vi "AutoWait.vi"(8 "error in (no error)":errorcluster, 11 "TimeOut (s)":dbl) -> (0 "error out":errorcluster)   [LabVIEW 2023]
doc: "Wrapper class for auto do nothing and wait\nInput:\n -- error in -- Cluster \n -- time out -- Double -- how long to wait B4 quitting\nOutput:\n -- error out -- Cluster"
uses:
  <vilib>/Rock Robotics/WPI/ThirdParty/JAS_Junk/TrajLib/ChassisSpeeds_New.vi
  <vilib>/Rock Robotics/WPI/ThirdParty/JAS_Junk/TrajLib/Conv_Feet_Meters.vi
  <vilib>/Rock Robotics/WPI/ThirdParty/JAS_Junk/TrajLib/Conv_Deg_Radians.vi
  <vilib>/Utility/semaphor.llb/Obtain Semaphore Reference.vi
  <vilib>/Rock Robotics/WPI/ThirdParty/JAS_Junk/TrajLib/Timer_Reset.vi
  Drive/DriveGlobal.vi
  <vilib>/Rock Robotics/WPI/ThirdParty/JAS_Junk/TrajLib/Trajectory_Library.lvlib
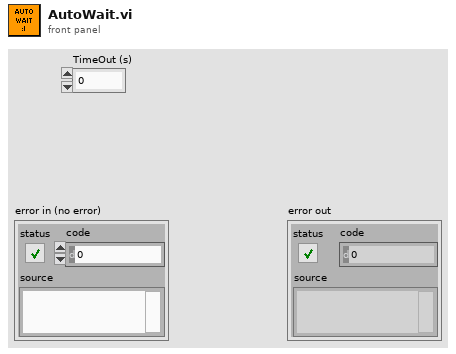
[diagram p1: front panel]
types:
  T1 = typedef "Trajectory_Library.lvlib/TIMER.ctl" = cluster{"StartTime":dbl, "Accumulated TIme":dbl, "Running":bool, "semaphore":T2}
  T2 = typedef "Semaphore RefNum" = refnum<k1>
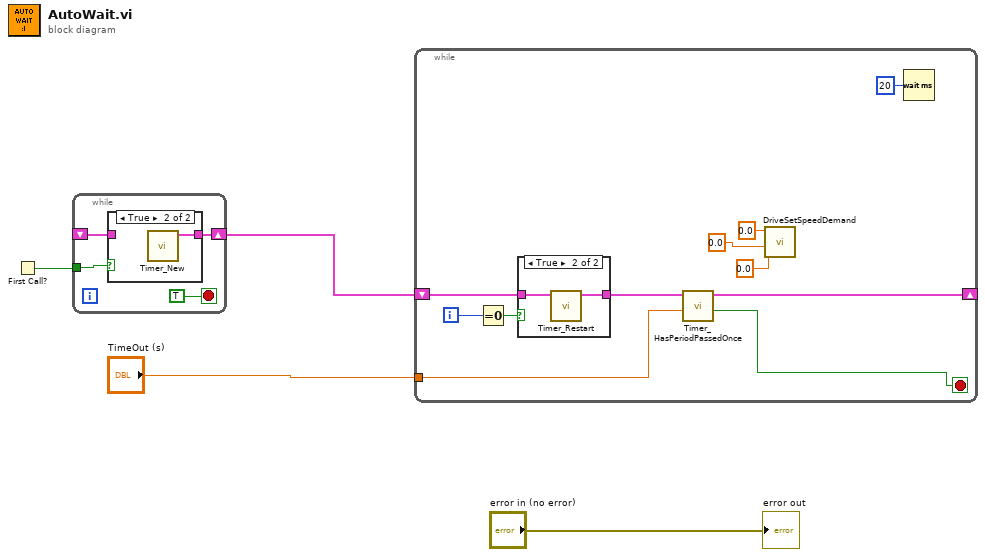
[diagram p0: block diagram]
diagram:
  n1 = First Call?() -> (First Call?: T/F=w2:bool)
  n2 = while {
    tunnel: w2 -> [w5]
    shift-right: [w8] -> w1
    shift-left: _ -> [w6]
    stop <- TRUE stop-if-true
    n3 = case shown="True" w5 {
      tunnel: [w9 w10] -> w8
      tunnel: w6 -> [w9 _]
      frame False {
      }
      frame True {
        n4 = call <vilib>:"Timer_New.vi"() -> ("TIMER"=w10:T1)  [unwired: 11 in]
      }
    }
  }
  n5 = while {
    tunnel: "TimeOut (s)" -> [w21]
    shift-right: [w15] -> _
    shift-left: w1 -> [w12]
    i -> [w14]
    stop <- w17 stop-if-true
    n6 = Equal To 0?(x=w14) -> (x = 0?=w13:bool)
    n7 = case shown="True" w13 {
      tunnel: w12 -> [w22 w24]
      tunnel: [w22 w23] -> w11
      frame False {
      }
      frame True {
        n8 = call <vilib>:"Timer_Restart.vi"("in Timer"=w24) -> ("out Timer"=w23:T1)  [unwired: 10 in]
      }
    }
    n9 = call <vilib>:"Timer_HasPeriodPassedOnce.vi"("Period"=w21, "in Timer"=w11) -> ("Expired"=w17:bool, "out Timer"=w15:T1)  [unwired: 7 in, 1 out]
    n10 = call "DriveSetSpeedDemand.vi"("ASpeedDemand (d/s)"=0.0 ("RSpeedDemand (ft/s)"), "YSpeedDemand (ft/s)"=0.0 ("RSpeedDemand (ft/s)"), "XSpeedDemand (ft/s)"=0.0 ("LSpeedDemand (ft/s)")) -> ()  [unwired: 9 in]
    n11 = Wait (ms)(milliseconds to wait=u32 20) -> ()  [unwired: 1 out]
  }
  "error out" <- "error in (no error)"
